vi "initialize.vi"(0 "HGF_Visitor":refnum<class "HGF_Visitor.lvclass">, 3 "initializationData":variant, 5 "error in (no error)":errorcluster, 7 "binaryString":string, 8 "I8 Array":i8[](array[numeric]), 9 "prependSize? (T)":bool, 11 "byteOrder (0:big-endian, network order)":T1(ring)) -> (14 "dup HGF_Visitor":refnum<class "HGF_Visitor.lvclass">, 17 "found?":bool, 19 "error out":errorcluster)   [LabVIEW 2014, in "HGF_BaseClasses.lvlib" / "HGF_Visitor.lvclass"]
doc: "This is a dynamic dispatch VI to be implemented by child classes to initialize their attributes.\n\n<B>Recommendation:</B> Use Variant for initialization data."
uses:
  HGF_Visitor.lvclass
  HGF_TriggeredEvent/HGF_TriggeredEvent.lvclass
  HGF_Base/HGF_Base.lvclass
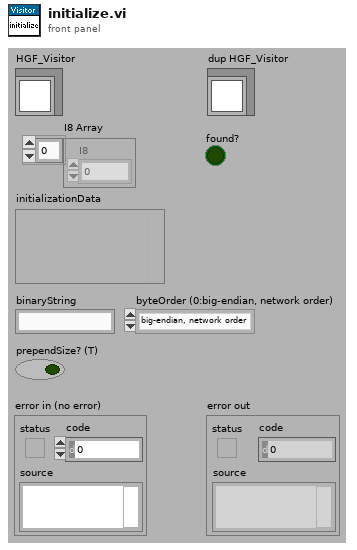
[diagram p1: front panel]
types:
  T1 = enum16{"big-endian, network order", "native, host order", "little-endian"}
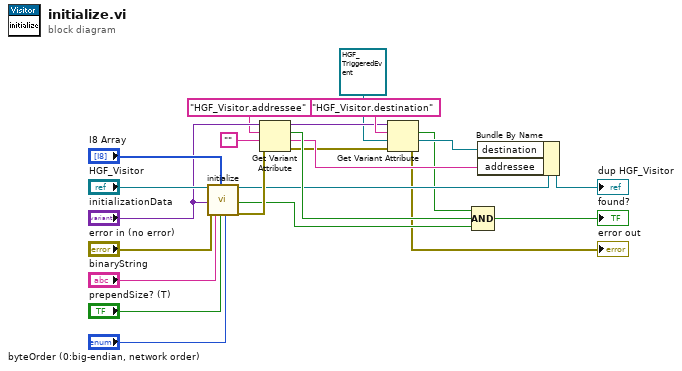
[diagram p0: block diagram]
diagram:
  n1 = call-parent "initialize.vi"("HGF_Base"="HGF_Visitor", "initializationData"="initializationData", "error in (no error)"="error in (no error)", "binaryString"="binaryString", "I8 Array"="I8 Array", "prependSize? (T)"="prependSize? (T)", "byteOrder (0:big-endian, network order)"="byteOrder (0:big-endian, network order)") -> ("dup HGF_Base"=w10:refnum<class "HGF_Visitor.lvclass">, "found?"=w12:bool, "error out"=w14:errorcluster)  [unwired: 10 out]
  n2 = Get Variant Attribute(Variant="initializationData", name="HGF_Visitor.addressee", default value (empty Variant)="", error in=w14) -> (duplicate Variant=w6:variant, found=w13:bool, value=w8:string, error out=w2:errorcluster)
  n3 = Get Variant Attribute(Variant=w6, name="HGF_Visitor.destination", default value (empty Variant)=refnum<class "HGF_TriggeredEvent.lvclass"> refnum ("HGF_BaseClasses.lvlib:HGF_TriggeredEvent.lvclass"), error in=w2) -> (found=w3:bool, value=w4:refnum<class "HGF_TriggeredEvent.lvclass">, error out=→"error out":errorcluster)  [unwired: 1 out]
  n4 = Compound Arithmetic op=AND(w3, w13, w12) -> (→"found?":bool)
  n5 = Bundle By Name(cluster=w10, "destination"=w4, "addressee"=w8) -> (→"dup HGF_Visitor":refnum<class "HGF_Visitor.lvclass">)
